vi "BRig_dataRT_stats__DAB_nTimeout.vi"() -> (2 "output_DAB_nTimeout":i32)   [LabVIEW 2014]
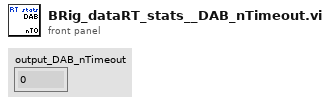
[diagram p1: front panel]
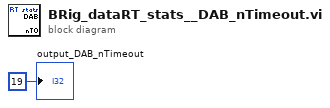
[diagram p0: block diagram]
diagram:
  "output_DAB_nTimeout" <- 19 ("output_iBlock")
